vi "Fetch IQ vs Slot Measurement Level.vi"(8 "error in (no error)":errorcluster, 10 "Instance (1)":i32=1 format="%.0g", 11 "VISA resource name":refnum<visa-resource-name>) -> (0 "error out":errorcluster, 1 "Results":dbl[](array[numeric]) format="%.2p", 2 "Reliability":i32, 3 "VISA resource name out":refnum<visa-resource-name>)   [LabVIEW 2020, in "Rohde&Schwarz CMXP GPRF.lvlib"]
doc: "Returns the averaged signal levels.\n\nAttribute:\nRSCMXPGPRF_ATTR_FETCH_IQ_VS_SLOT_MEASUREMENT_LEVEL\n\nRemote-control command:\nFETCh:GPRF:MEAS<i>:IQVSlot:LEVel?"
uses:
  <instrlib>/Rohde&Schwarz CMXP GPRF/Rohde&Schwarz CMXP GPRF.lvlib
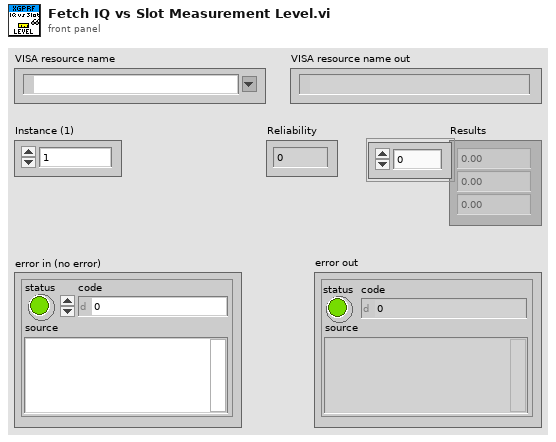
[diagram p1: front panel]
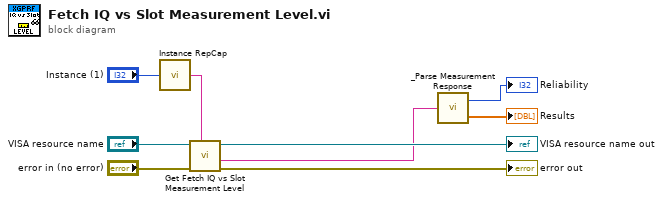
[diagram p0: block diagram]
diagram:
  n1 = call <instrlib>:"Instance RepCap.vi"("Instance in"="Instance (1)") -> ("Instance out"=w9:string)
  n2 = call "Get Fetch IQ vs Slot Measurement Level"("Repeated Capabilities"=w9, "error in (no error)"="error in (no error)", "instrument handle"="VISA resource name") -> ("error out"=→"error out":errorcluster, "Fetch IQ vs Slot Measurement Level"=w1:string, "instrument handle out"=→"VISA resource name out":refnum<visa-resource-name>)  [unwired: 6 in]
  n3 = call <instrlib>:"_Parse Measurement Response.vi"("String In"=w1) -> ("Reliability"=→"Reliability":i32, "Data"=→"Results":dbl[])
